vi "Handle Command.vi"(8 "error in":errorcluster, 10 "CMD in":refnum<class "Set Wvfm Write CMD.lvclass">, 11 "Object In":refnum<class>) -> (0 "error out":errorcluster, 1 "Command Successful?":bool, 2 "CMD out":refnum<class "Set Wvfm Write CMD.lvclass">, 3 "Object Out":refnum<class>)   [LabVIEW 2014, in "ePAS Library.lvlib" / "Set Wvfm Write CMD.lvclass"]
doc: "This VI will contain the code used to actually execute the request. If the request is successful, this will be indicated by the boolean output <b>Command Successful?</b>. The boolean output can then be used by the <b>Command Reply</b> which sends a reply if the reply queue is valid."
uses:
  Set Wvfm Write CMD.lvclass
  reusable/PAS/Main/PAS.lvclass
  reusable/PAS/Data/Main/PAS Data.lvclass
  reusable/Instrument/Instrument.lvclass/Instrument.ctl
  Set Wvfm Write CMD.lvclass/Set Wvfm Write CMD.ctl
  reusable/PAS/Data/Cell/PAS Cell Data.lvclass/PAS Cell Data.ctl
  reusable/PAS/Data/Cell/Write serializeWF_.vi
  reusable/Instrument/Read Data.vi
  reusable/Instrument/Write Data.vi
  reusable/PAS/Data/Main/Read CellData.vi
  reusable/PAS/Data/Main/Write CellData.vi
  reusable/Data/Data.lvclass
  reusable/PAS/Data/Cell/PAS Cell Data.lvclass
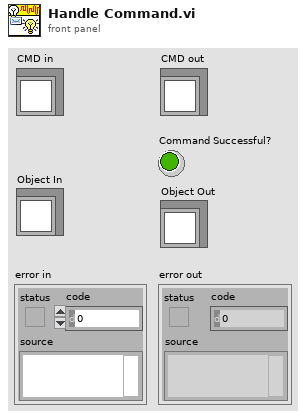
[diagram p1: front panel]
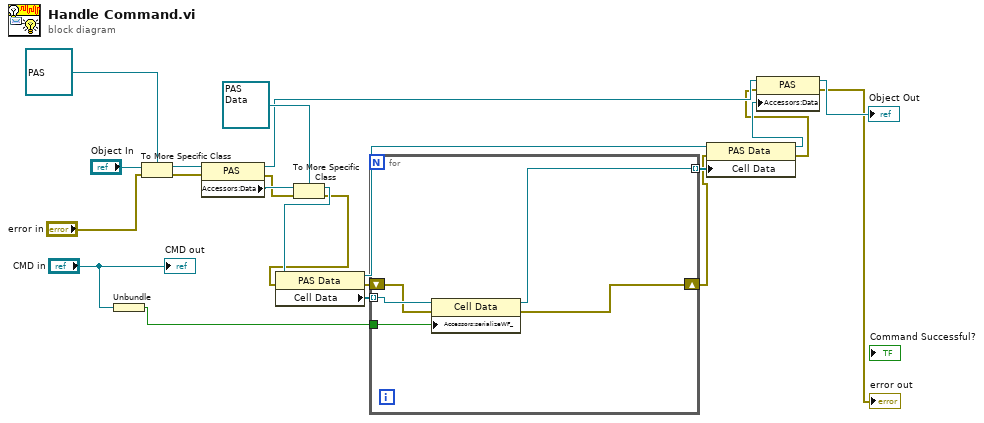
[diagram p0: block diagram]
diagram:
  n1 = Unbundle("CMD in") -> (w11:bool)
  n2 = To More Specific Class(target class=refnum<class "PAS.lvclass"> refnum ("PAS Library.lvlib:PAS"), reference="Object In", error in="error in") -> (specific class reference=w18:refnum<class "PAS.lvclass">, error out=w17:errorcluster)
  n3 = property class="PAS"(reference=w18, error in=w17) -> (reference out=w8:refnum<class "PAS.lvclass">, error out=w5:errorcluster, "Accessors:Data"=w16:refnum<class "Data.lvclass">)
  n4 = To More Specific Class(target class=refnum<class "PAS Data.lvclass"> refnum ("PAS Library.lvlib:PAS Data"), reference=w16, error in=w5) -> (specific class reference=w14:refnum<class "PAS Data.lvclass">, error out=w4:errorcluster)
  n5 = property class="PAS Data"(reference=w14, error in=w4) -> (reference out=w12:refnum<class "PAS Data.lvclass">, error out=w3:errorcluster, "Cell Data"=w13:refnum<class "PAS Cell Data.lvclass">[])
  n6 = for {
    tunnel: w13 -> [w27] mode=indexing
    tunnel: w11 -> [w26]
    tunnel: [w25] -> w10 mode=indexing
    shift-right: [w23] -> w2
    shift-left: w3 -> [w24]
    n7 = property class="Cell Data"(reference=w27, error in=w24, "Accessors:serializeWF_"=w26) -> (reference out=w25:refnum<class "PAS Cell Data.lvclass">, error out=w23:errorcluster)
  }
  n8 = property class="PAS Data"(reference=w12, error in=w2, "Cell Data"=w10) -> (reference out=w9:refnum<class "PAS Data.lvclass">, error out=w1:errorcluster)
  n9 = property class="PAS"(reference=w8, error in=w1, "Accessors:Data"=w9) -> (reference out=→"Object Out":refnum<class "PAS.lvclass">, error out=→"error out":errorcluster)
  "CMD out" <- "CMD in"
